vi "ReadDataAsRGB8Image.vi"(5 "alpha_channel_value":u8, 7 "Flip RB Channel Order":bool, 8 "error in (no error)":errorcluster, 11 "Buffer in":refnum<class "Buffer.lvclass">) -> (0 "error out":errorcluster, 3 "image":u32[][](array[numeric]))   [LabVIEW 2020, in "Buffer.lvclass"]
uses:
  Buffer.lvclass
  Buffer.lvclass/Buffer.ctl
  bin/gindustrialcam_32-1.dll
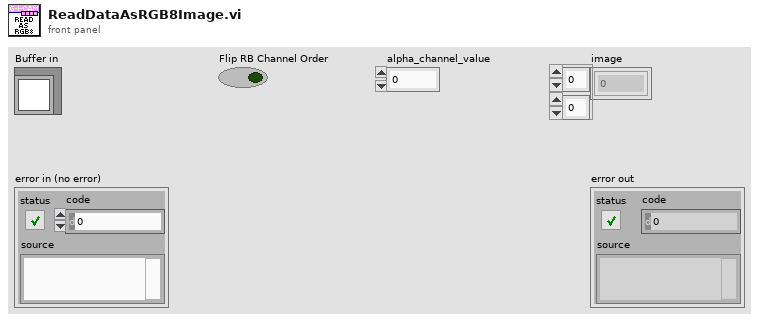
[diagram p1: front panel]
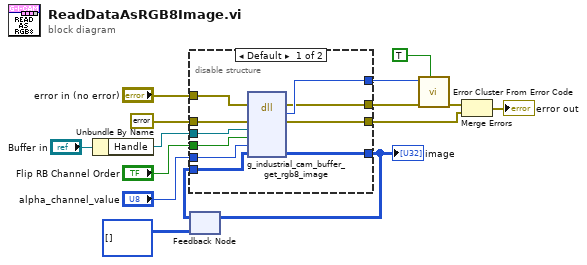
[diagram p0: block diagram]
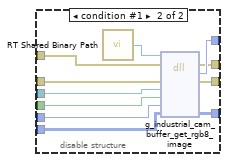
[diagram p2: hidden frame]
diagram:
  n1 = Unbundle By Name("Buffer in") -> ("Handle"=w5:refnum<data-value>)
  n2 = feedback #1(u32[][] [] ("Image")) -> (w7:u32[][])
  n3 = disable-structure shown="Default" {
    disable-tunnel: "Flip RB Channel Order" -> [w25 w36]
    disable-tunnel: [w24 w35] -> w14
    disable-tunnel: errorcluster {"status"=FALSE, "code"=0, "source"=""} ("error constant") -> [w23 w34]
    disable-tunnel: [w22 w33] -> w11
    disable-tunnel: [w21 w32] -> w9
    disable-tunnel: [w20 w31] -> w8
    disable-tunnel: w7 -> [w19 w30]
    disable-tunnel: w5 -> [w18 w29]
    disable-tunnel: "error in (no error)" -> [w17 w28]
    disable-tunnel: "alpha_channel_value" -> [w16 w27]
    frame condition #0 (active) {
      n4 = dll-call lib="C:/serenial/lib/g-industrial-camera/LabVIEW/g_industrial_cam/bin/gindustrialcam_*-1.*" fn="g_industrial_cam_buffer_get_rgb8_image"(error in=w17, "err"=w23, "edvr"=w18, "swap_rb_channels"=w25, "alpha_channel_value"=w16, "image"=w19) -> (error out=w20:errorcluster, "Mg_Error"=w21:i32, "err"=w22:errorcluster, "image"=w24:u32[][])  [unwired: 5 in, 1 out]
    }
    frame condition #1 {
      n5 = call "RT Shared Binary Path.vi"() -> ("Path"=w26:path)
      n6 = dll-call lib="C:/serenial/lib/g-industrial-camera/LabVIEW/g_industrial_cam/bin/gindustrialcam_*-1.*" fn="g_industrial_cam_buffer_get_rgb8_image"(path in=w26, error in=w28, "err"=w34, "edvr"=w29, "swap_rb_channels"=w36, "alpha_channel_value"=w27, "image"=w30) -> (error out=w31:errorcluster, "Mg_Error"=w32:i32, "err"=w33:errorcluster, "image"=w35:u32[][])  [unwired: 4 in, 1 out]
    }
  }
  "image" <- w14
  n7 = feedback-in #1(w14) -> ()
  n8 = call <vilib>:"Error Cluster From Error Code.vi"("show call chain? (False)"=TRUE, "error in (no error)"=w8, "error code (0)"=w9) -> ("error out"=w10:errorcluster)  [unwired: 6 in]
  n9 = Merge Errors(w10, w11) -> (→"error out":errorcluster)
